vi "Clear DUT.vi"(8 "error in (no error)":errorcluster, 11 "DUT Sample in":refnum<class "DUT Sample.lvclass">) -> (0 "error out":errorcluster)   [LabVIEW 2023, in "DUT Sample.lvclass"]
uses:
  DUT Sample.lvclass
  DUT Sample.lvclass/DUT Sample.ctl
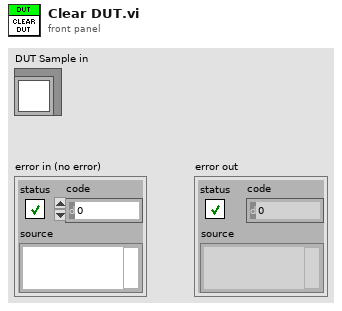
[diagram p1: front panel]
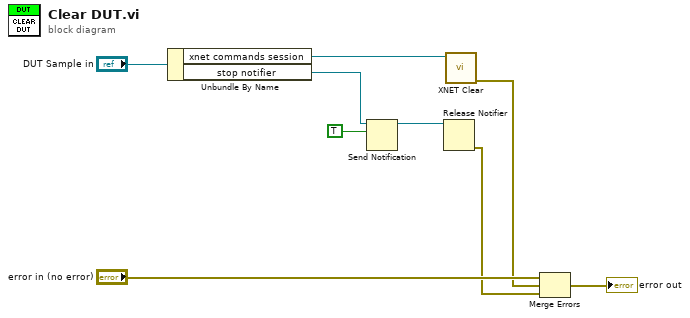
[diagram p0: block diagram]
diagram:
  n1 = Unbundle By Name("DUT Sample in") -> ("xnet commands session"=w8:refnum<k21>, "stop notifier"=w7:refnum<notifier>)
  n2 = Send Notification(notification=TRUE, notifier=w7) -> (notifier out=w5:refnum<notifier>)  [unwired: 1 in, 1 out]
  n3 = Release Notifier(notifier=w5) -> (error out=w2:errorcluster)  [unwired: 2 in, 2 out]
  n4 = call <vilib>:"XNET Clear.vi"("session in"=w8) -> ("error out"=w3:errorcluster)  [unwired: 14 in]
  n5 = Merge Errors("error in (no error)", w3, w2) -> (→"error out":errorcluster)
